vi "普通攻击动画.vi"() -> ()   [LabVIEW 2013]
panel:
  in  "簇":T1
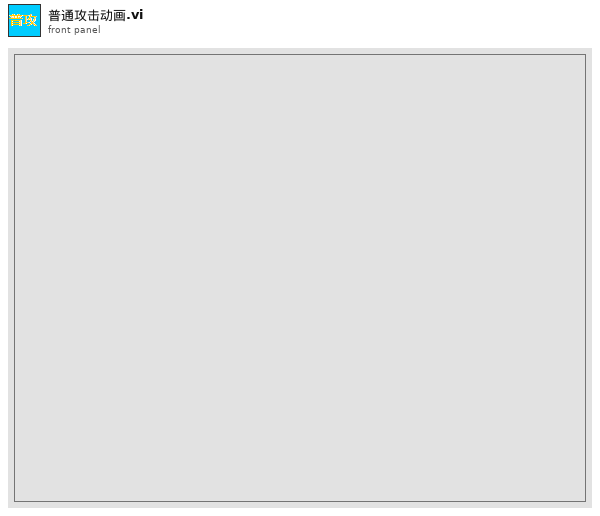
[diagram p1: front panel]
types:
  T1 = cluster{"1":bool, "2":bool, "3":bool, "4":bool, "5":bool, "6":bool, "7":bool, "8":bool, "9":bool, "减50":bool}
  T2 = cluster{"1":bool, "2":bool, "3":bool, "4":bool, "5":bool, "6":bool, "7":bool, "8":bool, "9":bool}
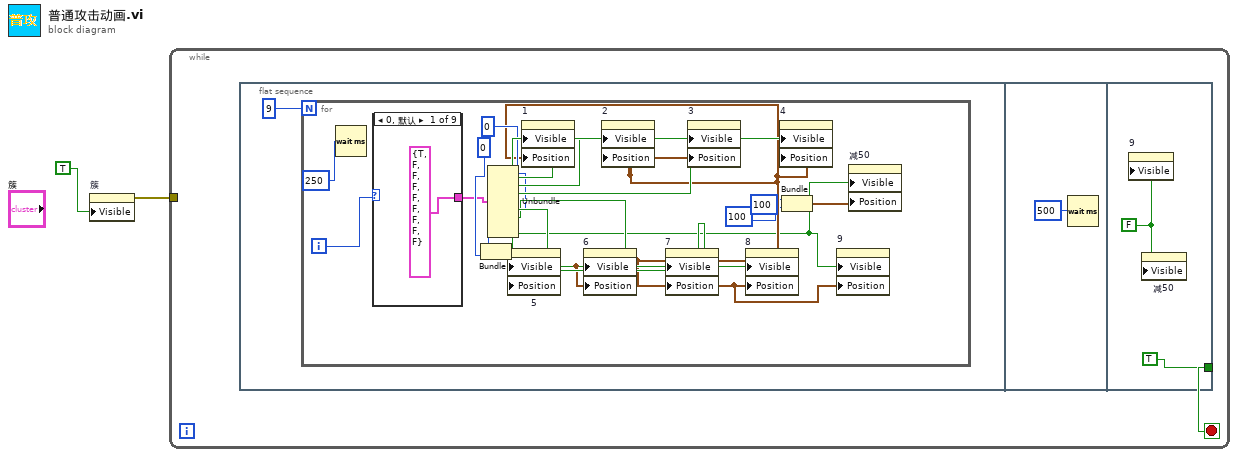
[diagram p0: block diagram]
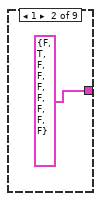
[diagram p2: hidden frame]
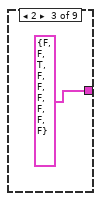
[diagram p3: hidden frame]
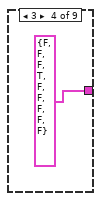
[diagram p4: hidden frame]
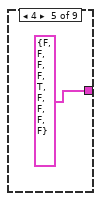
[diagram p5: hidden frame]
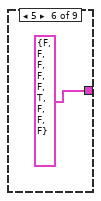
[diagram p6: hidden frame]
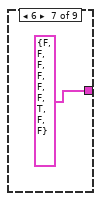
[diagram p7: hidden frame]
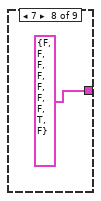
[diagram p8: hidden frame]
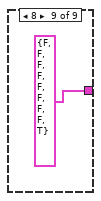
[diagram p9: hidden frame]
diagram:
  n1 = property on="簇" class="Clust"("Visible"=TRUE) -> (error out=w1:errorcluster)  [unwired: 2 in, 1 out]
  n2 = while {
    tunnel: w1 -> [_]
    stop <- w3 stop-if-true
    n3 = flat-sequence {
      tunnel: [TRUE] -> w3
      frame #0 {
        n4 = for {
          N: 9 -> [_]
          i -> [w11]
          n5 = Wait (ms)(milliseconds to wait=250) -> ()  [unwired: 1 out]
          n6 = case shown="0, 默认" w11 {
            tunnel: [T2 {"1"=TRUE, "2"=FALSE, "3"=FALSE, "4"=FALSE, "5"=FALSE, "6"=FALSE, "7"=FALSE, "8"=FALSE, "9"=FALSE} ("簇") T2 {"1"=FALSE, "2"=TRUE, "3"=FALSE, "4"=FALSE, "5"=FALSE, "6"=FALSE, "7"=FALSE, "8"=FALSE, "9"=FALSE} ("簇") T2 {"1"=FALSE, "2"=FALSE, "3"=TRUE, "4"=FALSE, "5"=FALSE, "6"=FALSE, "7"=FALSE, "8"=FALSE, "9"=FALSE} ("簇") T2 {"1"=FALSE, "2"=FALSE, "3"=FALSE, "4"=TRUE, "5"=FALSE, "6"=FALSE, "7"=FALSE, "8"=FALSE, "9"=FALSE} ("簇") T2 {"1"=FALSE, "2"=FALSE, "3"=FALSE, "4"=FALSE, "5"=TRUE, "6"=FALSE, "7"=FALSE, "8"=FALSE, "9"=FALSE} ("簇") T2 {"1"=FALSE, "2"=FALSE, "3"=FALSE, "4"=FALSE, "5"=FALSE, "6"=TRUE, "7"=FALSE, "8"=FALSE, "9"=FALSE} ("簇") T2 {"1"=FALSE, "2"=FALSE, "3"=FALSE, "4"=FALSE, "5"=FALSE, "6"=FALSE, "7"=TRUE, "8"=FALSE, "9"=FALSE} ("簇") T2 {"1"=FALSE, "2"=FALSE, "3"=FALSE, "4"=FALSE, "5"=FALSE, "6"=FALSE, "7"=FALSE, "8"=TRUE, "9"=FALSE} ("簇") T2 {"1"=FALSE, "2"=FALSE, "3"=FALSE, "4"=FALSE, "5"=FALSE, "6"=FALSE, "7"=FALSE, "8"=FALSE, "9"=TRUE} ("簇")] -> w10
            frame 0, Default {
            }
            frame 1 {
            }
            frame 2 {
            }
            frame 3 {
            }
            frame 4 {
            }
            frame 5 {
            }
            frame 6 {
            }
            frame 7 {
            }
            frame 8 {
            }
          }
          n7 = Bundle(0, 0) -> (w9:cluster{i32, i32})  [unwired: 1 in]
          n8 = Unbundle(w10) -> ("1"=w21:bool, "2"=w20:bool, "3"=w19:bool, "4"=w18:bool, "5"=w17:bool, "6"=w16:bool, "7"=w15:bool, "8"=w14:bool, "9"=w8:bool)
          n9 = property on="5" class="Bool"("Visible"=w17, "Position"=w9) -> ()  [unwired: 2 in, 2 out]
          n10 = property on="1" class="Bool"("Visible"=w21, "Position"=w9) -> ()  [unwired: 2 in, 2 out]
          n11 = property on="6" class="Bool"("Visible"=w16, "Position"=w9) -> ()  [unwired: 2 in, 2 out]
          n12 = property on="2" class="Bool"("Visible"=w20, "Position"=w9) -> ()  [unwired: 2 in, 2 out]
          n13 = property on="7" class="Bool"("Visible"=w15, "Position"=w9) -> ()  [unwired: 2 in, 2 out]
          n14 = property on="3" class="Bool"("Visible"=w19, "Position"=w9) -> ()  [unwired: 2 in, 2 out]
          n15 = property on="8" class="Bool"("Visible"=w14, "Position"=w9) -> ()  [unwired: 2 in, 2 out]
          n16 = property on="4" class="Bool"("Visible"=w18, "Position"=w9) -> ()  [unwired: 2 in, 2 out]
          n17 = Bundle(100, 100) -> (w5:cluster{i32, i32})  [unwired: 1 in]
          n18 = property on="9" class="Bool"("Visible"=w8, "Position"=w9) -> ()  [unwired: 2 in, 2 out]
          n19 = property on="减50" class="Bool"("Visible"=w8, "Position"=w5) -> ()  [unwired: 2 in, 2 out]
        }
      }
      frame #1 {
        n20 = Wait (ms)(milliseconds to wait=500) -> ()  [unwired: 1 out]
      }
      frame #2 {
        w34 = FALSE
        n21 = property on="9" class="Bool"("Visible"=w34) -> ()  [unwired: 2 in, 2 out]
        n22 = property on="减50" class="Bool"("Visible"=w34) -> ()  [unwired: 2 in, 2 out]
      }
    }
  }
